vi "Size.vi"(0 "State In":T1, 1 "XRef":refnum<vi>, 3 "Bounds":T3) -> (2 "State Out":T1, 4 "Reply":string[](array[string]))   [LabVIEW 2012, in "Unindex and Unbundle.xnode"]
doc: "This ability VI is called by LabVIEW after the user resizes the XNode. Bounds is a recatangle whose coordinates are given relative to the old top-left corner of the XNode. You must either return a UpdateImageAndBounds reply or not return anything, otherwise LabVIEW will generate an error. If you return UpdateImageAndBounds, you may also return other reply strings.\n\nDefault behavior: None.\n\nThis ability does not provide UI and OS messages are not handled.\n\nSee also: GetGrowInfo"
uses:
  Unindex and Unbundle.xnode
  State.ctl
  <vilib>/XNodeSupport/XNodeInt.ctl
  <vilib>/XNodeSupport/NI_XNodeSupport.lvlib
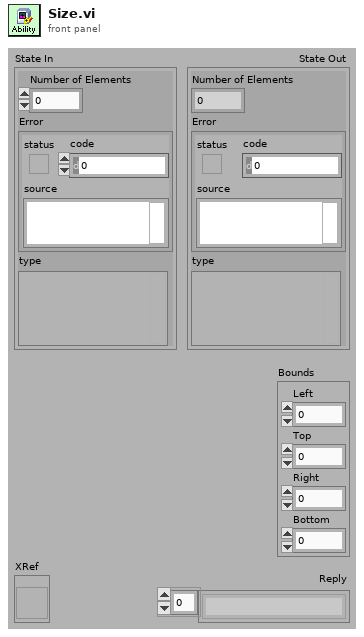
[diagram p1: front panel]
types:
  T1 = typedef "Unindex and Unbundle.xnode/State.ctl" = cluster{"Number of Elements":i32, "Error":errorcluster, "type":variant}
  T2 = typedef "NI_XNodeSupport.lvlib/XNodeInt.ctl" = i32
  T3 = cluster{"Left":T2, "Top":T2, "Right":T2, "Bottom":T2}
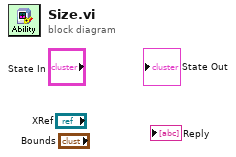
[diagram p0: block diagram]
diagram:
